vi "FYP_VI_MIDI_TableData.vi"(1 "input 2":u32, 2 "input 1":i16, 3 "array":string[][](array[string])) -> (0 "output array":string[][](array[string]))   [LabVIEW 2013]
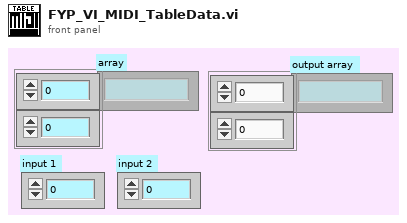
[diagram p1: front panel]
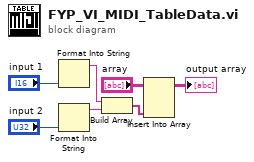
[diagram p0: block diagram]
diagram:
  n1 = Format Into String("input 1") -> (resulting string=w6:string)  [unwired: 3 in, 1 out]
  n2 = Format Into String("input 2") -> (resulting string=w7:string)  [unwired: 3 in, 1 out]
  n3 = Build Array(w6, w7) -> (w5:string[])
  n4 = Insert Into Array(array="array", new element=w5) -> (→"output array":string[][])  [unwired: 2 in]
